vi "Configure External Clock.vi"(0 "device session in":refnum<class "Device Session.lvclass">, 5 "external clock source":T1, 7 "external clock rate (Hz)":dbl=250000000.0 format="%#_6p", 11 "error in":errorcluster) -> (4 "device session out":refnum<class "Device Session.lvclass">, 6 "actual adc clock rate (Hz)":dbl=250000000.0 format="%#_6p", 15 "error out":errorcluster)   [LabVIEW 2015, in "Device Session.lvclass"]
doc: "Selects an external clock source and configures the external clock rate. When using an external clock, you must run the <B>Disable Data Clock</B> VI before disconnecting the external clock source.\n\n<B>Input Parameters</B>\n\n<B>device session in</B> is a reference to the session containing sessions to all instrument design libraries used in this sample project. This parameter is obtained from the 'Open Session' VI.\n\n<B>external clock source</B> specifies the source of the external clock.\n\n'Clock In' (default): specifies that the clock source is the Clock In signal from the device front panel.\n'PXIe DStar A': specifies that the clock source is the signal from the PXIe DStar A line.\n\n<B>external clock rate (Hz)</B> specifies the clock rate of the external clock. The default value is 250.\n\n<B>error in</B> describes error conditions that occur before this node runs. This input provides standard 'error in' functionality.\n\n<B>Output Parameters</B>\n\n<B>device session out</B> passes a reference to the session to the next VI.\n\n<B>actual adc clock rate (Hz)</B> returns coerced ADC clock rate in Hz.\n\n<B>error out</B> contains error information. This output provides standard 'error out' functionality."
uses:
  Device Session.lvclass
  <instrlib>/HSAI-RIO/Types/v1/Host/Typedefs/External Clock Source.ctl
  Device Session.lvclass/Device Session.ctl
  <instrlib>/HSAI-RIO/Config/Interface/v1/Host/Protected/Configure ADC Clock For External.vi
  <instrlib>/HSAI-RIO/Config/Interface/v1/Host/niHSAI Config v1 Host.lvclass
  <instrlib>/HSAI-RIO/Types/v1/Host/niHSAI Types v1 Host.lvlib
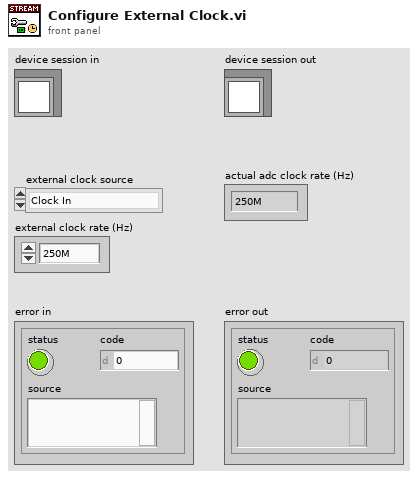
[diagram p1: front panel]
types:
  T1 = typedef "niHSAI Types v1 Host.lvlib/External Clock Source.ctl" = enum8{"Clock In", "PXIe DStar A"}
  T2 = typedef "Device Session.lvclass/Device Session Object.ctl" = cluster{"ni5171R FPGA Reference":T3, "niHSAI config":refnum<class "niHSAI Config v1 Host.lvclass">, "configured scaling coefficients":cluster{"gain":dbl, "offset":dbl}[], "number of channels to stream":u8, "selected acq channels":bool[], "number of channels":u32, "actual channel configuration":T4[], "configured channels":bool[], "sample clock rate (Hz)":dbl}
  T3 = typedef "Device Session.lvclass/FPGA Refnum.ctl" = refnum<k20>
  T4 = typedef "niHSAI Types v1 Host.lvlib/Channel Configuration.ctl" = cluster{"channel":u32, "coupling":T5, "impedance":T6, "bandwidth":T7, "vertical range":dbl, "vertical offset":dbl}
  T5 = typedef "niHSAI Types v1 Host.lvlib/Coupling.ctl" = enum8{"Default", "DC", "AC"}
  T6 = typedef "niHSAI Types v1 Host.lvlib/Impedance.ctl" = enum8{"Default", "1 mega ohm", "50 ohm"}
  T7 = typedef "niHSAI Types v1 Host.lvlib/Bandwidth.ctl" = enum8{"Default", "Full Bandwidth", "Anti-alias Filter"}
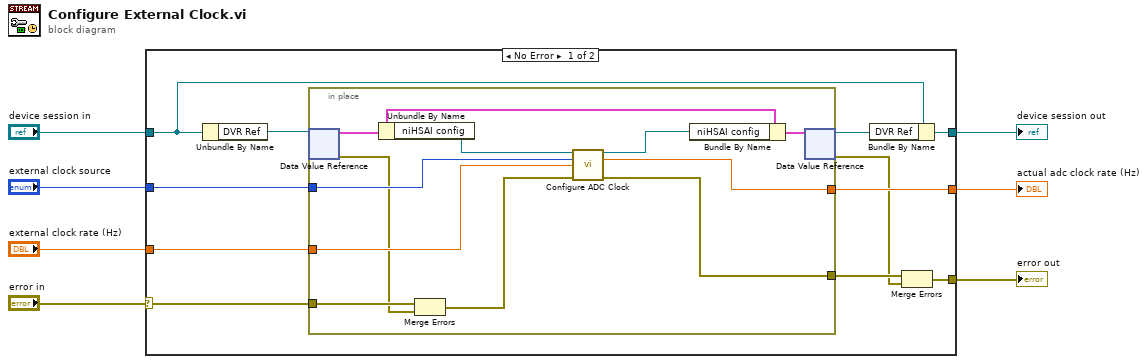
[diagram p0: block diagram]
diagram:
  n1 = case shown="No Error" "error in" {
    selector: "error in" -> [w18 w31]
    tunnel: "device session in" -> [w14 w30]
    tunnel: [w13 w30] -> w5
    tunnel: [w16 w31] -> w4
    tunnel: "external clock source" -> [w12 _]
    tunnel: "external clock rate (Hz)" -> [w11 _]
    tunnel: [w10 _] -> w1
    frame No Error {
      n2 = Unbundle By Name(w14) -> ("DVR Ref"=w15:refnum<data-value>)
      n3 = in-place {
        in-place-border: w18 -> [w20]
        in-place-border: [w29] -> w9
        in-place-border: w12 -> [w23]
        in-place-border: w11 -> [w22]
        in-place-border: [w21] -> w10
        n4 = in-place-dvr #1(w15) -> (w24:T2, w19:errorcluster)
        n5 = Unbundle By Name(w24) -> ("niHSAI config"=w26:refnum<class "niHSAI Config v1 Host.lvclass">)
        n6 = Merge Errors(w20, w19) -> (w27:errorcluster)
        n7 = call-poly <instrlib>:"Configure ADC Clock.vi"("session in"=w26, "external clock source"=w23, "external clock rate (Hz)"=w22, "error in"=w27) -> ("session out"=w28:refnum<class "niHSAI Config v1 Host.lvclass">, "actual adc clock rate (Hz)"=w21:dbl, "error out"=w29:errorcluster)  [unwired: 8 in, 1 out]
        n8 = Bundle By Name(cluster=w24, "niHSAI config"=w28) -> (w25:T2)
        n9 = in-place-dvr #1(w25) -> (w17:refnum<data-value>, w8:errorcluster)
      }
      n10 = Bundle By Name(cluster=w14, "DVR Ref"=w17) -> (w13:refnum<class "Device Session.lvclass">)
      n11 = Merge Errors(w9, w8) -> (w16:errorcluster)
    }
    frame Error {
    }
  }
  "error out" <- w4
  "device session out" <- w5
  "actual adc clock rate (Hz)" <- w1
